vi "Dequeue with Exit.vi"(8 "error in (no error)":errorcluster, 11 "Queue In":refnum<queue>) -> (0 "error out":errorcluster, 1 "Data":variant, 2 "State":T1, 3 "Queue Out":refnum<queue>, 5 "Exit":bool)   [LabVIEW 2013, in "VI Internal QSM.lvlib"]
uses:
  VI Internal QSM.lvlib
  UserDefined Control/QSM Msg.ctl
  UserDefined Control/QSM State.ctl
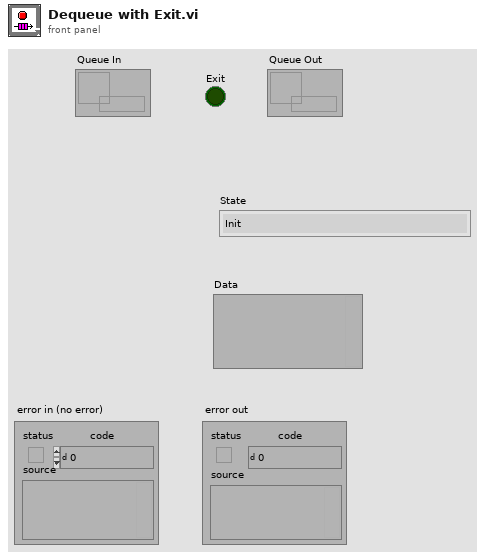
[diagram p1: front panel]
types:
  T1 = typedef "VI Internal QSM.lvlib/QSM State.ctl" = enum16{"Init", "Idle", "Error", "Exit", "Test"}
  T2 = typedef "VI Internal QSM.lvlib/QSM Msg.ctl" = cluster{"State":T1, "Data":variant}
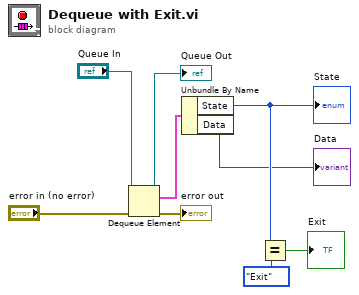
[diagram p0: block diagram]
diagram:
  n1 = Dequeue Element(queue="Queue In", error in (no error)="error in (no error)") -> (queue out=→"Queue Out":refnum<queue>, element=w6:T2, error out=→"error out":errorcluster)  [unwired: 1 in, 1 out]
  n2 = Unbundle By Name(w6) -> ("State"=w4:T1, "Data"=→"Data":variant)
  "State" <- w4
  n3 = Equal?(x=w4, y=QSM_State."Exit" ("State")) -> (x = y?=→"Exit":bool)
